vi "Get FIFOs.vi"(6 "offset":i32, 8 "error in (no error)":errorcluster, 10 "DMA channel visibility filter":T4, 11 "bitfile xml in":string) -> (0 "error out":errorcluster, 2 "DMA configuration array":T1[](array[typedef]), 4 "offset past EndTag":i32)   [LabVIEW 2010, in "FPGA Bitfile Utility.lvlib"]
uses:
  <userlib>/_FPGA Interface Advanced Tools/FPGA Bitfile Utility/FPGA Bitfile Utility.lvlib
  <vilib>/rvi/ClientSDK/Host Interface/DMA/public/niFpgaDmaChannelVisibilityFilter.ctl
  <vilib>/rvi/FIFO/Fifo_Types/Fifo_DMA_Config.ctl
  <vilib>/rvi/DataTransferAndStorage/Container/Common/niFpgaDataTypeControl.ctl
  <vilib>/rvi/ClientSDK/Core/ModuleGeneration/CommunicationInterfaceUtility/niFpgaDmaChannelImplementation.ctl
  <vilib>/rvi/Utilities/XML/nirviXML_GetValue_String.vi
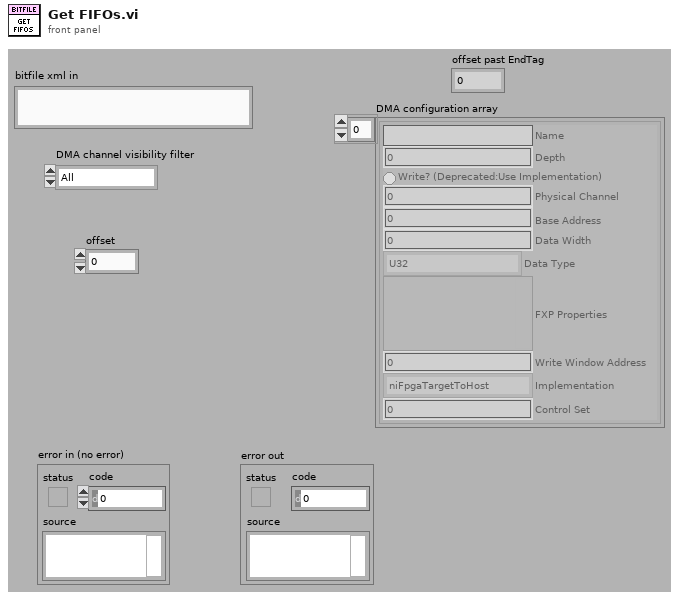
[diagram p1: front panel]
types:
  T1 = typedef "Fifo_DMA_Config.ctl" = cluster{"Name":string, "Depth":u32, "Write? (Deprecated:Use Implementation)":bool, "Physical Channel":u32, "Base Address":u32, "Data Width":u32, "Data Type":T2, "FXP Properties":variant, "Write Window Address":u32, "Implementation":T3, "Control Set":u32}
  T2 = typedef "niFpgaDataTypeControl.ctl" = enum32{"Boolean", "I8", "I16", "I32", "I64", "U8", "U16", "U32", "U64", "FXP", "CustomControl"}
  T3 = typedef "niFpgaDmaChannelImplementation.ctl" = enum16{"niFpgaTargetToHost", "niFpgaHostToTarget", "niFpgaPeerToPeerWriter", "niFpgaPeerToPeerReader", "niCoreTargetToHost", "niCoreHostToTarget"}
  T4 = typedef "niFpgaDmaChannelVisibilityFilter.ctl" = enum16{"All", "UserVisible"}
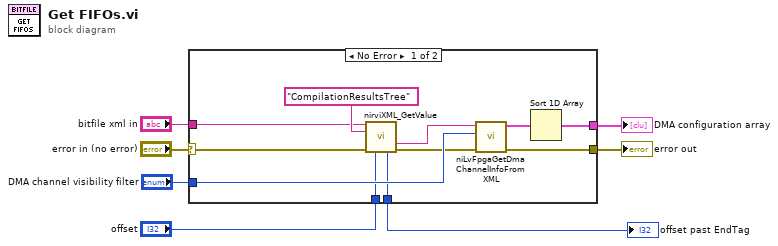
[diagram p0: block diagram]
diagram:
  n1 = case shown="No Error" "error in (no error)" {
    selector: "error in (no error)" -> [w14 w20]
    tunnel: [w18 _] -> w4
    tunnel: [w17 w20] -> w5
    tunnel: "DMA channel visibility filter" -> [w15 _]
    tunnel: "offset" -> [w10 w19]
    tunnel: [w9 w19] -> w2
    tunnel: "bitfile xml in" -> [w8 _]
    frame No Error {
      n2 = call-poly <vilib>:"nirviXML_GetValue.vi"("xml string in"=w8, "tag name in"="CompilationResultsTree" ("tag"), "error in (no error)"=w14, "offset"=w10) -> ("value"=w12:string, "offset past EndTag"=w9:i32, "error out"=w13:errorcluster)  [unwired: 1 in, 8 out]
      n3 = call "niLvFpgaGetDmaChannelInfoFromXML.vi"("error in (no error)"=w13, "DMA Channel Filter"=w15, "XML String in"=w12) -> ("error out"=w17:errorcluster, "DMA configuration array"=w16:T1[])  [unwired: 7 out]
      n4 = Sort 1D Array(array=w16) -> (sorted array=w18:T1[])
    }
    frame Error {
    }
  }
  "DMA configuration array" <- w4
  "error out" <- w5
  "offset past EndTag" <- w2
